vi "NMF.vi"(8 "error in":errorcluster) -> (0 "error out":errorcluster, 3 "out":refnum<class "NMF.lvclass">)   [LabVIEW 2020]
doc: "Non-Negative Matrix Factorization (NMF).\n\n Find two non-negative matrices (W, H) whose product approximates the non-\n negative matrix X. This factorization can be used for example for\n dimensionality reduction, source separation or topic extraction.\n\n The objective function is:\n\n .. math::\n\n 0.5 * ||X - WH||_{loss}^2 + alpha * l1_{ratio} * ||vec(W)||_1\n\n + alpha * l1_{ratio} * ||vec(H)||_1\n\n + 0.5 * alpha * (1 - l1_{ratio}) * ||W||_{Fro}^2\n\n + 0.5 * alpha * (1 - l1_{ratio}) * ||H||_{Fro}^2\n\n Where:\n\n :math:`||A||_{Fro}^2 = \\sum_{i,j} A_{ij}^2` (Frobenius norm)\n\n :math:`||vec(A)||_1 = \\sum_{i,j} abs(A_{ij})` (Elementwise L1 norm)\n\n The generic norm :math:`||X - WH||_{loss}` may represent\n the Frobenius norm or another supported beta-divergence loss.\n The choice between options is controlled by the `beta_loss` parameter.\n\n The objective function is minimized with an alternating minimization of W\n and H.\n\n Read more in the :ref:`User Guide <NMF>`.\n\n Parameters\n ----------\n n_components : int, default=None\n Number of components, if n_components is not set all features\n are kept.\n\n init : {'random', 'nndsvd', 'nndsvda', 'nndsvdar', 'custom'}, default=None\n Method used to initialize the procedure.\n Default: None.\n Valid options:\n\n - `None`: 'nndsvd' if n_components <= min(n_samples, n_features),\n otherwise random.\n\n - `'random'`: non-negative random matrices, scaled with:\n sqrt(X.mean() / n_components)\n\n - `'nndsvd'`: Nonnegative Double Singular Value Decomposition (NNDSVD)\n initialization (better for sparseness)\n\n - `'nndsvda'`: NNDSVD with zeros filled with the average of X\n (better when sparsity is not desired)\n\n - `'nndsvdar'` NNDSVD with zeros filled with small random values\n (generally faster, less accurate alternative to NNDSVDa\n for when sparsity is not desired)\n\n - `'custom'`: use custom matrices W and H\n\n solver : {'cd', 'mu'}, default='cd'\n Numerical solver to use:\n 'cd' is a Coordinate Descent solver.\n 'mu' is a Multiplicative Update solver.\n\n .. versionadded:: 0.17\n Coordinate Descent solver.\n\n .. versionadded:: 0.19\n Multiplicative Update solver.\n\n beta_loss : float or {'frobenius', 'kullback-leibler', 'itakura-saito'}, default='frobenius'\n Beta divergence to be minimized, measuring the distance between X\n and the dot product WH. Note that values different from 'frobenius'\n (or 2) and 'kullback-leibler' (or 1) lead to significantly slower\n fits. Note that for beta_loss <= 0 (or 'itakura-saito'), the input\n matrix X cannot contain zeros. Used only in 'mu' solver.\n\n .. versionadded:: 0.19\n\n tol : float, default=1e-4\n Tolerance of the stopping condition.\n\n max_iter : int, default=200\n Maximum number of iterations before timing out.\n\n random_state : int, RandomState instance or None, default=None\n Used for initialisation (when ``init`` == 'nndsvdar' or\n 'random'), and in Coordinate Descent. Pass an int for reproducible\n results across multiple function calls.\n See :term:`Glossary <random_state>`.\n\n alpha : float, default=0.\n Constant that multiplies the regularization terms. Set it to zero to\n have no regularization.\n\n .. versionadded:: 0.17\n *alpha* used in the Coordinate Descent solver.\n\n l1_ratio : float, default=0.\n The regularization mixing parameter, with 0 <= l1_ratio <= 1.\n For l1_ratio = 0 the penalty is an elementwise L2 penalty\n (aka Frobenius Norm).\n For l1_ratio = 1 it is an elementwise L1 penalty.\n For 0 < l1_ratio < 1, the penalty is a combination of L1 and L2.\n\n .. versionadded:: 0.17\n Regularization parameter *l1_ratio* used in the Coordinate Descent\n solver.\n\n verbose : int, default=0\n Whether to be verbose.\n\n shuffle : bool, default=False\n If true, randomize the order of coordinates in the CD solver.\n\n .. versionadded:: 0.17\n *shuffle* parameter used in the Coordinate Descent solver.\n\n regularization : {'both', 'components', 'transformation', None}, default='both'\n Select whether the regularization affects the components (H), the\n transformation (W), both or none of them.\n\n .. versionadded:: 0.24\n\n Attributes\n ----------\n components_ : ndarray of shape (n_components, n_features)\n Factorization matrix, sometimes called 'dictionary'.\n\n n_components_ : int\n The number of components. It is same as the `n_components` parameter\n if it was given. Otherwise, it will be same as the number of\n features.\n\n reconstruction_err_ : float\n Frobenius norm of the matrix difference, or beta-divergence, between\n the training data ``X`` and the reconstructed data ``WH`` from\n the fitted model.\n\n n_iter_ : int\n Actual number of iterations.\n\n \nAvailable methods:\nFit\nFit Transform\nTransform\nGet Attributes\nGet Params\nSet Params"
uses:
  NMF.lvclass
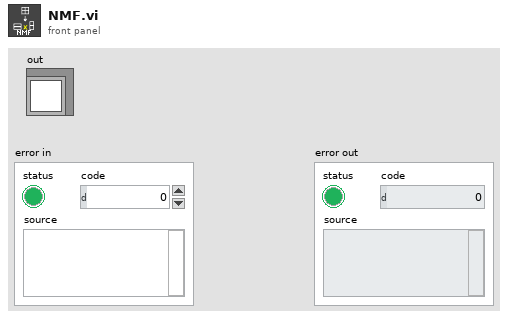
[diagram p1: front panel]
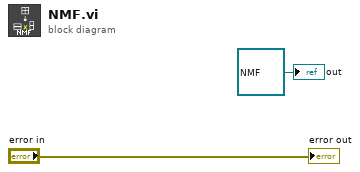
[diagram p0: block diagram]
diagram:
  "out" <- refnum<class "NMF.lvclass"> refnum ("model")
  "error out" <- "error in"
